vi "CLFNWrapperCallGateway.vi"(8 "error in (no error)":errorcluster, 11 "appended path":path) -> (0 "error out":errorcluster, 2 "ref":i32, 3 "path out":path)   [LabVIEW 2011]
doc: "Execution system set to standard to prevent this DLL from loading in UI thread, which causes labview hang"
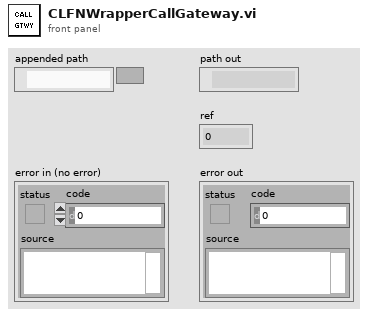
[diagram p1: front panel]
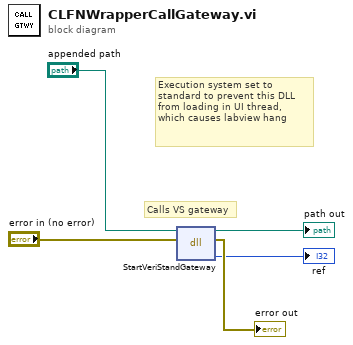
[diagram p0: block diagram]
diagram:
  # "Execution system set to standard to prevent this DLL from loading in UI thread, which causes labview hang"
  # "Calls VS gateway"
  n1 = dll-call lib="C:/Program Files (x86)/National Instruments/VeriStand 2010/Data/NationalInstruments.VeriStand.Gateway.dll" fn="StartVeriStandGateway"(path in="appended path", error in="error in (no error)") -> (path out=→"path out":path, error out=→"error out":errorcluster, "ref"=→"ref":i32)  [unwired: 3 in]
